vi "IsValid.vi"(1 "context in":refnum<class "Context.lvclass">) -> (0 "valid?":bool)   [LabVIEW 2025, in "ZeroMQ.lvlib" / "Context.lvclass"]
doc: "Checks whether the supplied context object is valid"
uses:
  Context.lvclass
  Context.lvclass/Context.ctl
panel:
  # "ØMQ"
  # "labview"
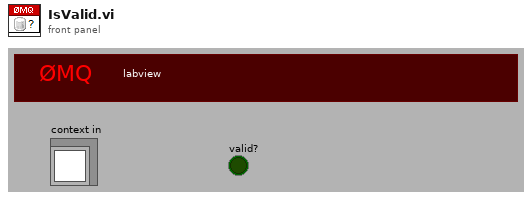
[diagram p1: front panel]
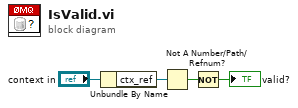
[diagram p0: block diagram]
diagram:
  n1 = Unbundle By Name("context in") -> ("ctx_ref"=w3:refnum<data-value>)
  n2 = Not A Number/Path/Refnum?(number/path/refnum=w3) -> (NaN/Path/Refnum?=w2:bool)
  n3 = Not(x=w2) -> (.not. x?=→"valid?":bool)
